vi "auto_chopper.vi"(8 "error in (no error)":errorcluster, 9 "chopper params":T1, 10 "y arr":dbl[](array[numeric]), 11 "x arr":dbl[](array[numeric])) -> (0 "error out":errorcluster, 2 "y arr possibly chopped":dbl[](array[numeric]), 3 "x arr possibly chopped":dbl[](array[numeric]), 4 "max index(es)":i32, 5 "entire Y":dbl[](graph), 6 "min index(es)":i32, 7 "entire x":dbl[](graph))   [LabVIEW 2016]
uses:
  ctl/Chopper Parameters -- Cluster.ctl
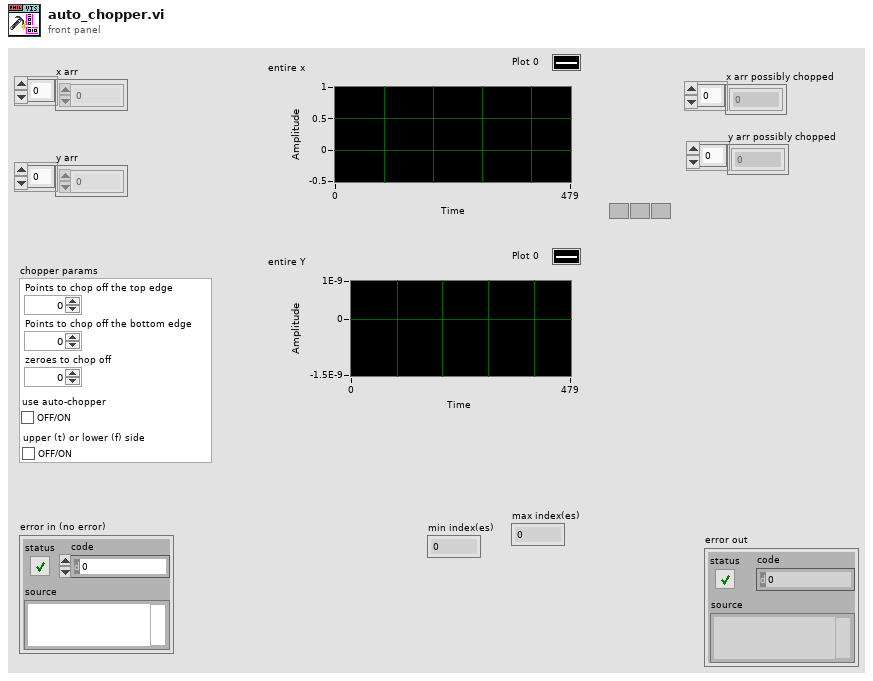
[diagram p1: front panel]
types:
  T1 = typedef "Chopper Parameters -- Cluster.ctl" = cluster{"Points to chop off the top edge":i32, "Points to chop off the bottom edge":i32, "zeroes to chop off":i32, "use auto-chopper":bool, "upper (t) or lower (f) side":bool}
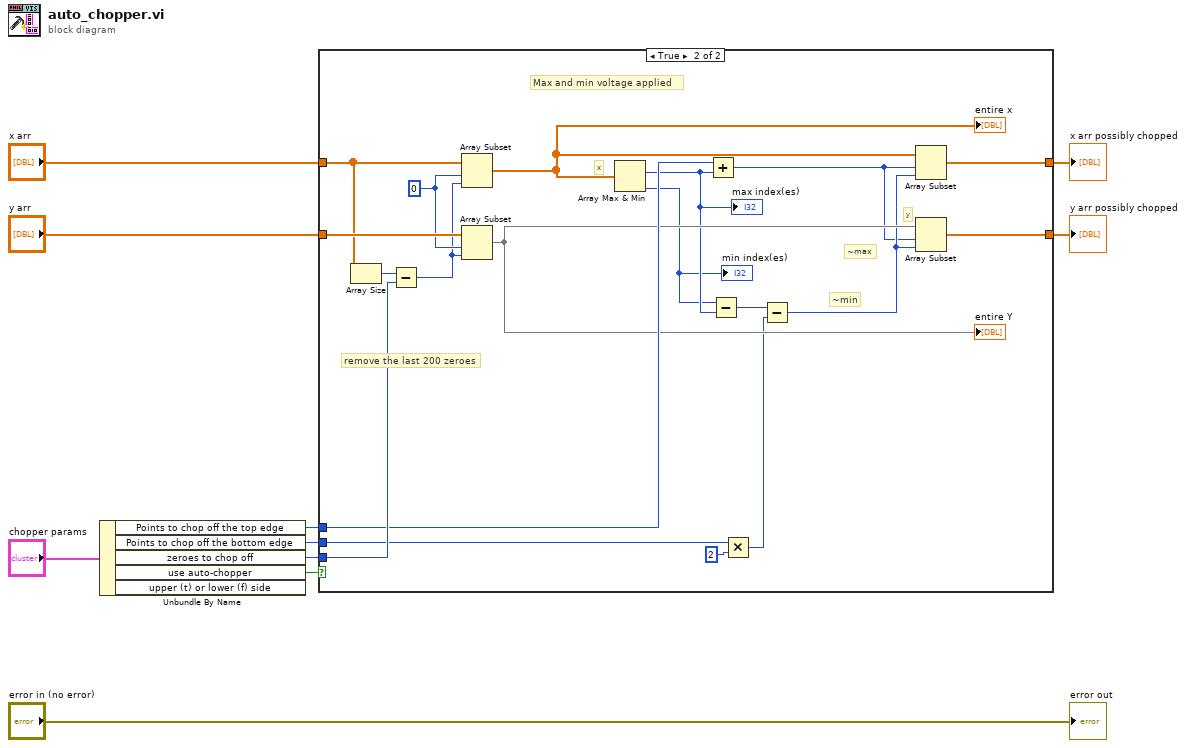
[diagram p0: block diagram]
diagram:
  n1 = Unbundle By Name("chopper params") -> ("Points to chop off the top edge"=w8:i32, "Points to chop off the bottom edge"=w9:i32, "zeroes to chop off"=w10:i32, "use auto-chopper"=w5:bool)  [unwired: 1 out]
  n2 = case shown="True" w5 {
    tunnel: w10 -> [_ w31]
    tunnel: w9 -> [_ w30]
    tunnel: w8 -> [_ w29]
    tunnel: "y arr" -> [w11 w28]
    tunnel: "x arr" -> [w12 w27]
    tunnel: [w11 w16] -> w4
    tunnel: [w12 w15] -> w3
    frame False {
    }
    frame True {
      w24 = 0 ("index")
      # "~min"
      # "~max"
      # "y"
      # "x"
      # "remove the last 200 zeroes"
      # "Max and min voltage applied"
      n3 = Array Size(array=w27) -> (size(s)=w22:i32)
      n4 = Subtract(x=w22, y=w31) -> (x-y=w23:i32)
      n5 = Array Subset(array=w27, index=w24, length=w23) -> (w25:dbl[])
      "entire x" <- w25
      n6 = Array Subset(array=w28, index=w24, length=w23) -> (w26:dbl[])
      "entire Y" <- w26
      n7 = Array Max & Min(array=w25) -> (max index (indices)=w18:i32, min index (indices)=w17:i32)  [unwired: 2 out]
      "max index(es)" <- w18
      "min index(es)" <- w17
      n8 = Add(x=w29, y=w18) -> (x+y=w13:i32)
      n9 = Subtract(x=w17, y=w18) -> (x-y=w19:i32)
      n10 = Multiply(x=w30, y=2) -> (x*y=w21:i32)
      n11 = Subtract(x=w19, y=w21) -> (x-y=w14:i32)
      n12 = Array Subset(array=w25, index=w13, length=w14) -> (w15:dbl[])
      n13 = Array Subset(array=w26, index=w13, length=w14) -> (w16:dbl[])
    }
  }
  "x arr possibly chopped" <- w3
  "y arr possibly chopped" <- w4
  "error out" <- "error in (no error)"
